vi "removeEdge.vi"(0 "reference":refnum<class "NoteNode.lvclass">, 1 "graph":refnum<class "Graph.lvclass">, 2 "edge":refnum<class "AbstractEdge.lvclass">, 5 "error in (no error)":errorcluster) -> (14 "reference out":refnum<class "NoteNode.lvclass">, 19 "error out":errorcluster)   [LabVIEW 2016, in "NoteNode.lvclass"]
doc: "public void removeEdge(Graph g, Edge e)"
uses:
  <resource>/Framework/Providers/Open_GDS/UML/NoteNode_class/NoteNode.lvclass
  <resource>/Framework/Providers/Open_GDS/UML/Graph_class/Graph.lvclass
  <resource>/Framework/Providers/Open_GDS/UML/AbstractEdge_class/AbstractEdge.lvclass
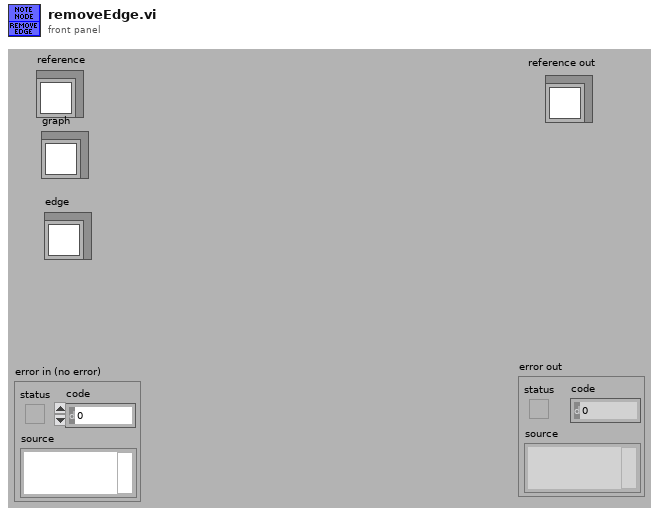
[diagram p1: front panel]
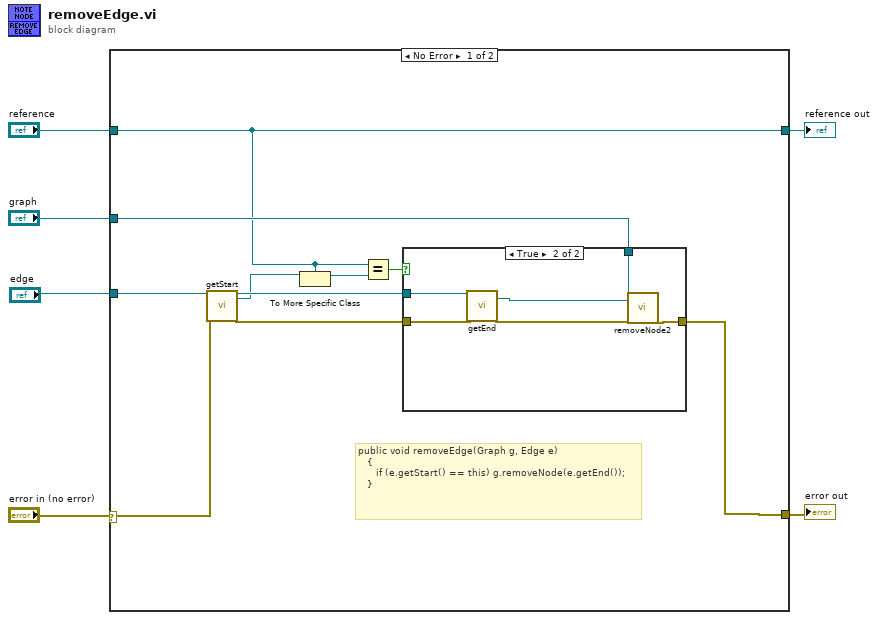
[diagram p0: block diagram]
diagram:
  n1 = case shown="No Error" "error in (no error)" {
    selector: "error in (no error)" -> [w15 w24]
    tunnel: "reference" -> [w7 w25]
    tunnel: [w16 w24] -> w5
    tunnel: [w7 w25] -> w4
    tunnel: "edge" -> [w14 _]
    tunnel: "graph" -> [w13 _]
    frame No Error {
      # "public void removeEdge(Graph g, Edge e)\n   {\n      if (e.getStart() == this) g.removeNode(e.getEnd());\n   }"
      n2 = call-dynamic "getStart.vi"("reference"=w14, "error in (no error)"=w15) -> ("reference out"=w10:refnum<class "AbstractEdge.lvclass">, "startNode"=w9:refnum<class "AbstractNode.lvclass">, "error out"=w11:errorcluster)  [unwired: 14 in, 1 out]
      n3 = To More Specific Class(target class=w7, reference=w9) -> (specific class reference=w8:refnum<class "NoteNode.lvclass">)  [unwired: 1 in, 1 out]
      n4 = Equal?(x=w7, y=w8) -> (x = y?=w12:bool)
      n5 = case shown="True" w12 {
        tunnel: w11 -> [w17 w23]
        tunnel: w13 -> [_ w18]
        tunnel: w10 -> [_ w22]
        tunnel: [w17 w21] -> w16
        frame False {
        }
        frame True {
          n6 = call-dynamic "getEnd.vi"("reference"=w22, "error in (no error)"=w23) -> ("endNode"=w19:refnum<class "AbstractNode.lvclass">, "error out"=w20:errorcluster)  [unwired: 14 in, 2 out]
          n7 = call-dynamic "removeNode2.vi"("reference"=w18, "node"=w19, "error in (no error)"=w20) -> ("error out"=w21:errorcluster)  [unwired: 15 in, 1 out]
        }
      }
    }
    frame Error {
    }
  }
  "reference out" <- w4
  "error out" <- w5
